vi "filtro_Instru.vi"   [LabVIEW 2014]
uses:
  <vilib>/Analysis/NI_AALBase.lvlib
  <vilib>/Analysis/3filter.llb/IIR Filter (DBL).vi
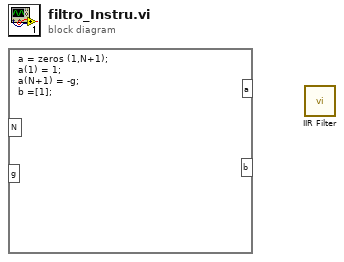
[diagram p0: block diagram]
diagram:
  n1 = formula code="a = zeros (1,N+1);\na(1) = 1; \na(N+1) = -g;\nb =[1];"() -> ()  [unwired: 2 in, 2 out]
  n2 = call-poly <vilib>:"IIR Filter.vi"() -> ()  [unwired: 4 in, 2 out]
